vi "PDP Loop.vi"() -> ()   [LabVIEW 2016]
uses:
  Common Code/PDP Status Cluster.ctl
  Robot Global Data.vi
panel:
  out "all currents (A)":dbl[](array[numeric])
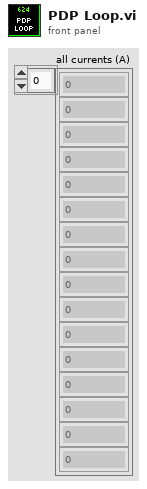
[diagram p1: front panel]
types:
  T1 = typedef "PDP Status Cluster.ctl" = cluster{"Drivetrain Left CIM 1":dbl, "Drivetrain Left CIM 2":dbl, "Drivetrain Left Mini CIM":dbl, "Drivetrain Right CIM 1":dbl, "Drivetrain Right CIM 2":dbl, "Drivetrain Right Mini CIM":dbl, "Drivetrain Center CIM 1":dbl, "Drivetrain Center CIM 2":dbl, "Shooter Motor 1":dbl, "Shooter Motor 2":dbl, "Climber Motor 1":dbl, "Climber Motor 2":dbl, "Intake Motor":dbl, "Trigger Motor":dbl, "Fans/Compressor":dbl}
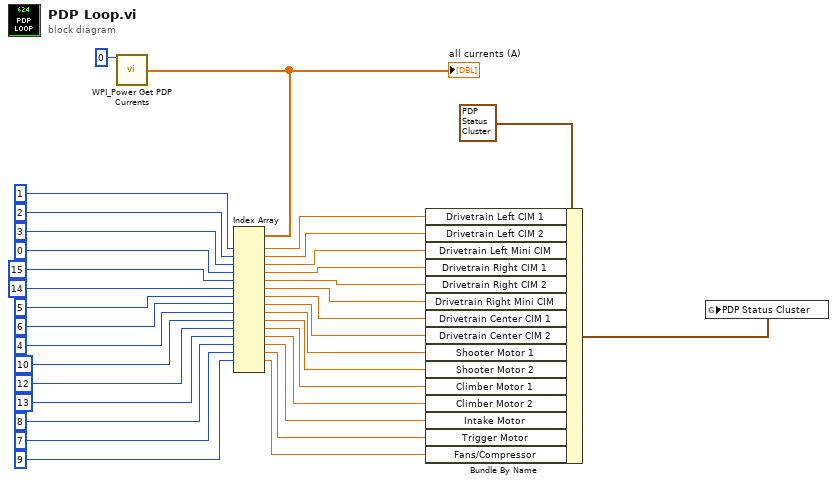
[diagram p0: block diagram]
diagram:
  n1 = call <vilib>:"WPI_Power Get PDP Currents.vi"("Power Distribution Panel (0)"=u8 0) -> ("all currents (A)"=w34:dbl[])  [unwired: 12 in, 2 out]
  "all currents (A)" <- w34
  n2 = Index Array(array=w34, index #1=1, index #2=2, index #3=3, index #4=0, index #5=15, index #6=14, index #7=5, index #8=6, index #9=4, index #10=10, index #11=12, index #12=13, index #13=8, index #14=7, index #15=9) -> (element #1=w30:dbl, element #2=w29:dbl, element #3=w28:dbl, element #4=w27:dbl, element #5=w26:dbl, element #6=w25:dbl, element #7=w24:dbl, element #8=w23:dbl, element #9=w1:dbl, element #10=w22:dbl, element #11=w21:dbl, element #12=w20:dbl, element #13=w19:dbl, element #14=w18:dbl, element #15=w17:dbl)  [unwired: 1 in, 1 out]
  n3 = Bundle By Name(cluster=T1 {"Drivetrain Left CIM 1"=0.0, "Drivetrain Left CIM 2"=0.0, "Drivetrain Left Mini CIM"=0.0, "Drivetrain Right CIM 1"=0.0, "Drivetrain Right CIM 2"=0.0, "Drivetrain Right Mini CIM"=0.0, "Drivetrain Center CIM 1"=0.0, "Drivetrain Center CIM 2"=0.0, "Shooter Motor 1"=0.0, "Shooter Motor 2"=0.0, "Climber Motor 1"=0.0, "Climber Motor 2"=0.0, "Intake Motor"=0.0, "Trigger Motor"=0.0, "Fans/Compressor"=0.0} ("PDP Status Cluster"), "Drivetrain Left CIM 1"=w30, "Drivetrain Left CIM 2"=w29, "Drivetrain Left Mini CIM"=w28, "Drivetrain Right CIM 1"=w27, "Drivetrain Right CIM 2"=w26, "Drivetrain Right Mini CIM"=w25, "Drivetrain Center CIM 1"=w24, "Drivetrain Center CIM 2"=w23, "Shooter Motor 1"=w1, "Shooter Motor 2"=w22, "Climber Motor 1"=w21, "Climber Motor 2"=w20, "Intake Motor"=w19, "Trigger Motor"=w18, "Fans/Compressor"=w17) -> (w31:T1)
  n4 = global write "Robot Global Data.vi" "PDP Status Cluster"(w31) -> ()
